vi "AVS_PrepareMeasure.vi"(0 "a_hDevice":i32, 7 "MeasConfArray":u8[](array[numeric])) -> (4 "Output Value":i32)   [LabVIEW 2020]
uses:
  AvaSpecX64-DLL_9.4/avaspecx64.dll
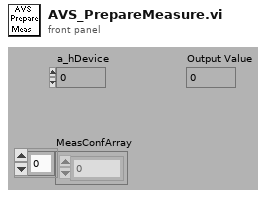
[diagram p1: front panel]
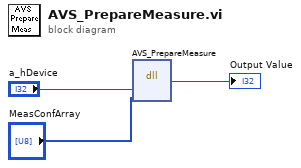
[diagram p0: block diagram]
diagram:
  n1 = dll-call lib="C:/AvaSpecX64-DLL_9.4/avaspecx64.dll" fn="AVS_PrepareMeasure"("a_hDevice"="a_hDevice", "MeasConfArray"="MeasConfArray") -> ("return type"=→"Output Value":i32)  [unwired: 5 in, 2 out]
